vi "brake_test.vi"() -> ()   [LabVIEW 2018]
uses:
  <vilib>/Platform/TimedLoop/XDataNode/timing_clust.ctl
  <vilib>/Platform/TimedLoop/XDataNode/nitl_modes.ctl
  <vilib>/Platform/TimedLoop/XDataNode/wakeup.ctl
  <vilib>/rvi/Emulation/niFpgaGetClockAttributes.vi
  <vilib>/rvi/Emulation/niFpgaSctlEmulationGetInTimedLoop.vi
  <vilib>/rvi/Emulation/niFpgaEmulationReportErrorSimple.vi
  <vilib>/rvi/Emulation/niFpgaProcessEmulError.vi
  <vilib>/rvi/Emulation/niFpgaCriticalErrorInLSC.vi
  <vilib>/Platform/TimedLoop/XDataNode/XDataNode.xnode
  <vilib>/Platform/TimedLoop/XDataNode/XDNodeRunTimeDep.lvlib
panel:
  in  "drain":bool
  in  "brake_2":bool=TRUE
  in  "brake_1":bool=TRUE
  out "fxp_P_lp2":i32
  out "fxp_P_lp1":i32
  out "fxp_P_hp2":i32
  out "fxp_P_hp1":i32
  out "drain_valve_state":bool
  out "brake_state":bool
  in  "stop":bool
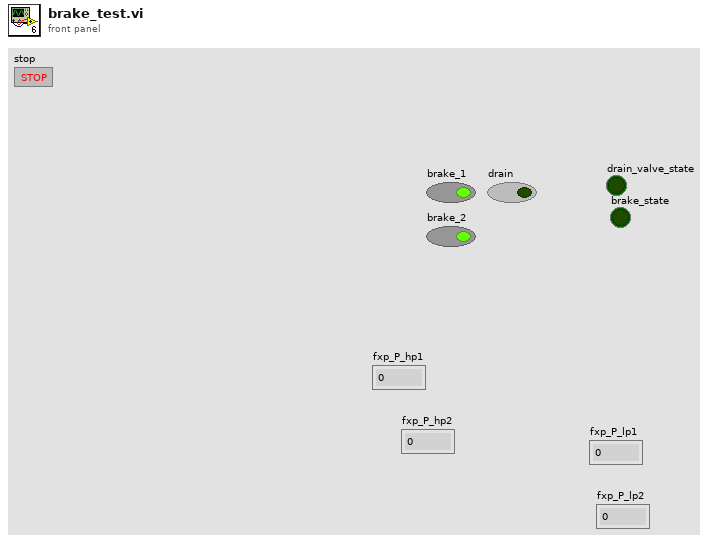
[diagram p1: front panel]
types:
  T1 = typedef "XDNodeRunTimeDep.lvlib/timing_clust.ctl" = cluster{"Expected End [f-1]":u64, "Actual End [f-1]":u64, "Finished Late? [f-1]":bool, "Expected End [i-1]":u64, "Actual End [i-1]":u64, "Finished Late? [i-1]":bool, "Expected Start [i]":u64, "Actual Start [i]":u64, "Expected Start [f]":u64, "Actual Start [f]":u64, "Source Name":string, "Structure Name":string, "Period":i64, "Deadline":i64, "Offset":i64, "Start":i64, "Priority":i32, "Timeout":i32, "Mode":T2, "Wakeup Reason":T3, "Error":errorcluster, "Source Type":string, "Secondary Source Type":string, "Global End Time":u64, "Global Start Time":u64, "Frame Duration":u64, "Iteration Duration":u64, "Assigned CPU":i32, "I/O Scan Engine Mode":u32}
  T2 = typedef "XDNodeRunTimeDep.lvlib/nitl_modes.ctl" = enum32{"No Change", "Process missed periods, maintain original phase", "Discard missed periods, maintain original phase", "Process missed periods, ignore original phase", "Discard missed periods, ignore original phase"}
  T3 = typedef "XDNodeRunTimeDep.lvlib/wakeup.ctl" = enum32{"Normal", "Aborted", "Asynchronous wakeup", "Timing source error", "Timed loop error", "Timeout"}
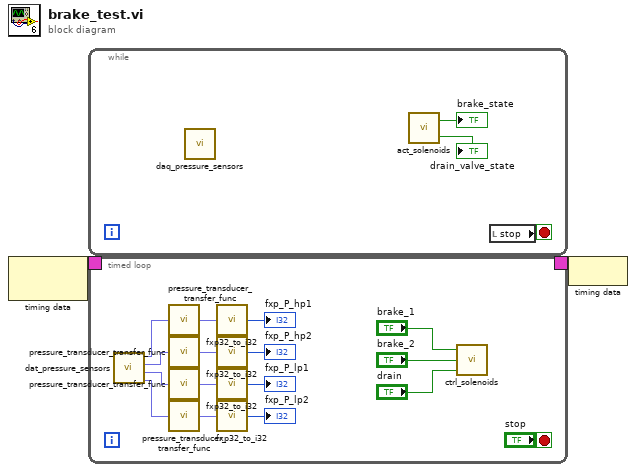
[diagram p0: block diagram]
diagram:
  n1 = node-c288() -> (w2:T1)  [unwired: 1 in]
  n2 = while {
    stop <- w5 stop-if-true
    n3 = call "daq_pressure_sensors.vi"() -> ()  [unwired: 2 in]
    n4 = call "act_solenoids.vi"() -> ("drain_valve_state"=→"drain_valve_state":bool, "brake_state"=→"brake_state":bool)  [unwired: 2 in]
    n5 = local read "stop"() -> (w5:bool)
  }
  n6 = timed-loop {
    timing: w2 -> [_]
    timing-out: [_] -> w1
    stop <- "stop" stop-if-true
    n7 = call "dat_pressure_sensors.vi"() -> ("P_lp2"=w9:fxp<+/-,24,5>, "P_lp1"=w10:fxp<+/-,24,5>, "P_hp2"=w11:fxp<+/-,24,5>, "P_hp1"=w12:fxp<+/-,24,5>)  [unwired: 8 in]
    n8 = call "pressure_transducer_transfer_func.vi"("p_v"=w12) -> ("pressure"=w20:fxp<+/-,32,16>)
    n9 = call "pressure_transducer_transfer_func.vi"("p_v"=w11) -> ("pressure"=w18:fxp<+/-,32,16>)
    n10 = call "pressure_transducer_transfer_func.vi"("p_v"=w10) -> ("pressure"=w16:fxp<+/-,32,16>)
    n11 = call "pressure_transducer_transfer_func.vi"("p_v"=w9) -> ("pressure"=w14:fxp<+/-,32,16>)
    n12 = call "fxp32_to_i32.vi"("fxp32_16"=w20) -> ("32bit integer"=→"fxp_P_hp1":i32)
    n13 = call "fxp32_to_i32.vi"("fxp32_16"=w18) -> ("32bit integer"=→"fxp_P_hp2":i32)
    n14 = call "fxp32_to_i32.vi"("fxp32_16"=w16) -> ("32bit integer"=→"fxp_P_lp1":i32)
    n15 = call "fxp32_to_i32.vi"("fxp32_16"=w14) -> ("32bit integer"=→"fxp_P_lp2":i32)
    n16 = call "ctrl_solenoids.vi"("drain"="drain", "brake_2"="brake_2", "brake_1"="brake_1") -> ()
  }
  n17 = node-c288(w1) -> ()
